vi "Folder Creater.vi"(8 "error in (no error)":errorcluster, 10 "Variant name":string, 11 "dup path in":path) -> (0 "error out":errorcluster, 3 "dup path out":path)   [LabVIEW 2017]
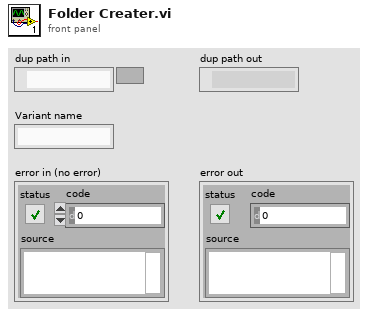
[diagram p1: front panel]
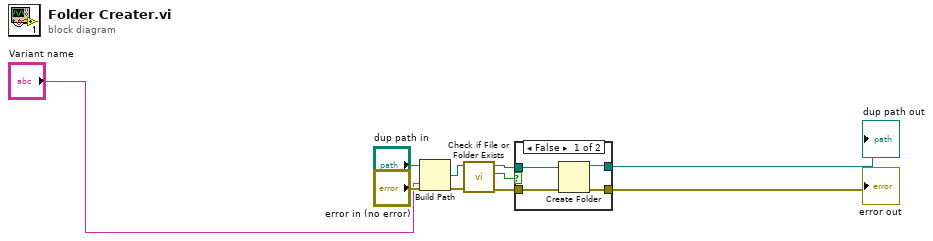
[diagram p0: block diagram]
diagram:
  n1 = Build Path(base path="dup path in", name or relative path="Variant name") -> (appended path=w3:path)
  n2 = call <vilib>:"Check if File or Folder Exists.vi"("error in (no error)"="error in (no error)", "path"=w3) -> ("error out"=w6:errorcluster, "file or folder exists?"=w5:bool, "dup path"=w4:path)  [unwired: 7 in]
  n3 = case shown="False" w5 {
    tunnel: w4 -> [w13 w15]
    tunnel: w6 -> [w12 w14]
    tunnel: [w11 w15] -> w8
    tunnel: [w10 w14] -> w9
    frame False {
      n4 = Create Folder(path (use dialog)=w13, error in=w12) -> (created path=w11:path, error out=w10:errorcluster)  [unwired: 1 in, 1 out]
    }
    frame True {
    }
  }
  "error out" <- w9
  "dup path out" <- w8
